vi "MainServer.vi"() -> ()   [LabVIEW 2012]
uses:
  <vilib>/addons/database/Connection.llb/DB Tools Open Connec (Path).vi
  <vilib>/addons/database/NI_Database_API.lvlib
panel:
  out "error":i32[](array[numeric])
  out "length":i32[](array[numeric])
  in  "Port":u16=1721
  out "# of Connections":i32
  in  "stop":bool
  in  "listen halted":bool
  out "Array":string[](array[string])
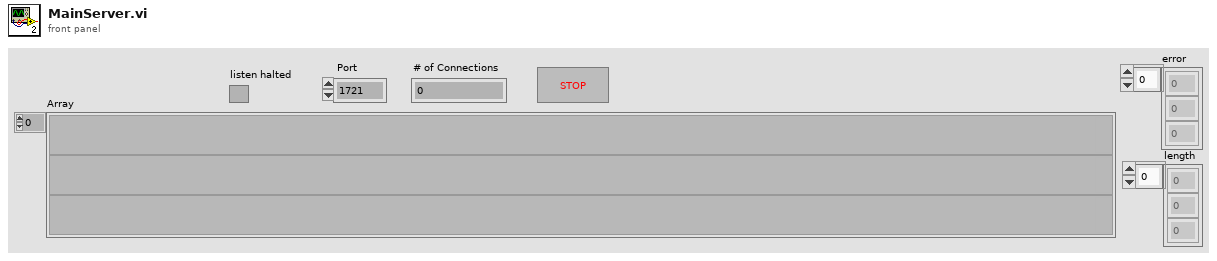
[diagram p1: front panel]
types:
  T1 = typedef "NI_Database_API.lvlib/Conn ObjectReference.ctl" = refnum<k1>
  T2 = enum16{"Standard", "Buffered", "CRLF", "Immediate"}
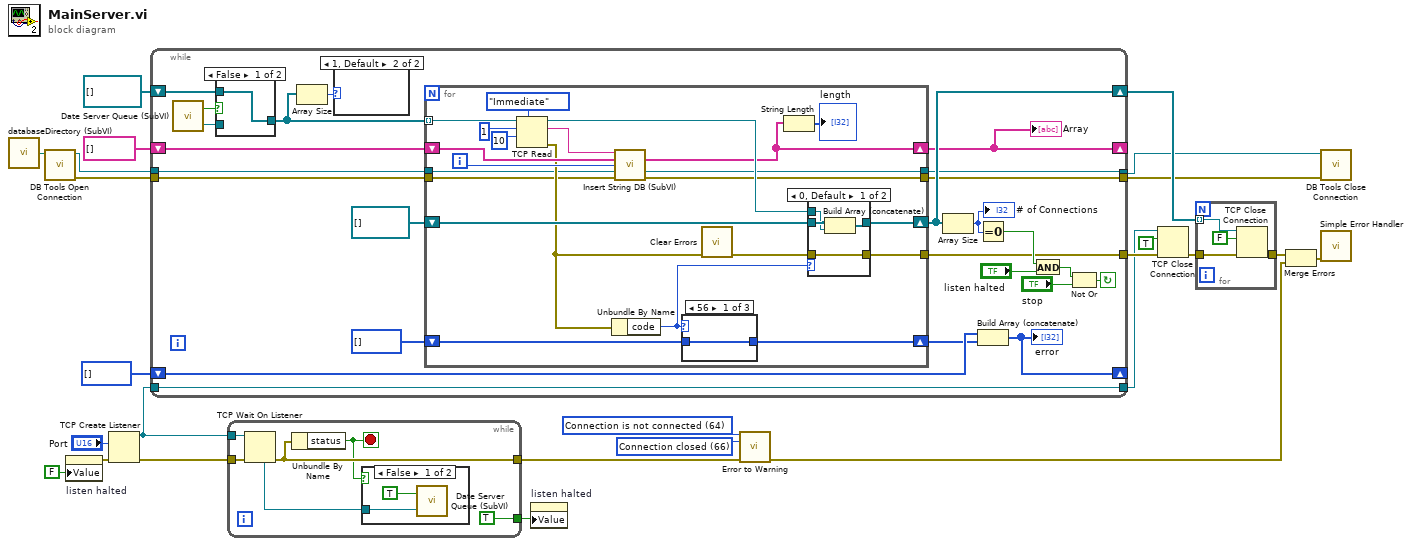
[diagram p0: block diagram]
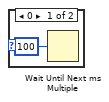
[diagram p2: hidden frame]
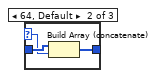
[diagram p3: hidden frame]
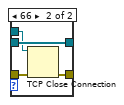
[diagram p5: hidden frame]
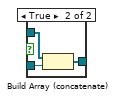
[diagram p6: hidden frame]
diagram:
  w18 = 66 items=["No Error", "Argument Error", "Memory Full", "Out of Zone", "End of File", "File Already Open", "Generic File IO Error", "File Not Found", "File Permission Error", "Disk Full", "Duplicate Path", "Too Many Files Open", "Not Enabled", "Resource File Not Found", "Cannot Add Resource", "Resource Not Found", "Image Not Found", "Image Memory Error", "Pen Does Not Exist", "Config Bad Type", "Config Token Not Found", "Config Parse Error", "Config Memory Error", "Bad External Code Format", "Bad External Code Offset", "External Code Not Present", "Null Window", "Destroy Window Mixup", "Null Menu", "Print Aborted", "Bad Print Record", "Print Driver Error", "Windows Error During Print", "Memory Error During Print", "Print Dialog Error", "Generic Print Error", "Invalid Device Refnum", "Device Not Found", "Device Parameter Error", "Device Unit Error", "Can't Open Device", "Device Call Aborted", "Generic Error", "Cancelled By User", "Object ID Too Low", "Object ID Too High", "Object Not In Heap", "Unknown Heap", "Bad DefProc ID", "DefProc Not In Table", "Message Out Of Range", "Null Method", "Unknown Message", "Manager Call Not Supported", "Bad address", "Connection In progress", "Connection timed out", "Connection is already in progress", "Network attribute not supported", "Network error", "Address in use", "System out of memory", "Connection aborted", "Connection refused", "Connection is not connected", "Connection is already connected", "Connection closed", "Initialize error (interapplication manager)", "Bad occurrence", "Wait on unbound occurrence handler", "Occurrence queue overflow", "Bad path", "Semaphore not signaled", "Unrecognized type (interapplication manager)"] ("2nd Error to Convert")
  w19 = 64 items=["No Error", "Argument Error", "Memory Full", "Out of Zone", "End of File", "File Already Open", "Generic File IO Error", "File Not Found", "File Permission Error", "Disk Full", "Duplicate Path", "Too Many Files Open", "Not Enabled", "Resource File Not Found", "Cannot Add Resource", "Resource Not Found", "Image Not Found", "Image Memory Error", "Pen Does Not Exist", "Config Bad Type", "Config Token Not Found", "Config Parse Error", "Config Memory Error", "Bad External Code Format", "Bad External Code Offset", "External Code Not Present", "Null Window", "Destroy Window Mixup", "Null Menu", "Print Aborted", "Bad Print Record", "Print Driver Error", "Windows Error During Print", "Memory Error During Print", "Print Dialog Error", "Generic Print Error", "Invalid Device Refnum", "Device Not Found", "Device Parameter Error", "Device Unit Error", "Can't Open Device", "Device Call Aborted", "Generic Error", "Cancelled By User", "Object ID Too Low", "Object ID Too High", "Object Not In Heap", "Unknown Heap", "Bad DefProc ID", "DefProc Not In Table", "Message Out Of Range", "Null Method", "Unknown Message", "Manager Call Not Supported", "Bad address", "Connection In progress", "Connection timed out", "Connection is already in progress", "Network attribute not supported", "Network error", "Address in use", "System out of memory", "Connection aborted", "Connection refused", "Connection is not connected", "Connection is already connected", "Connection closed", "Initialize error (interapplication manager)", "Bad occurrence", "Wait on unbound occurrence handler", "Occurrence queue overflow", "Bad path", "Semaphore not signaled", "Unrecognized type (interapplication manager)"] ("1st Error to Convert")
  n1 = call "databaseDirectory (SubVI).vi"() -> ("Application Directory"=w1:path)  [unwired: 1 in]
  n2 = call-poly <vilib>:"DB Tools Open Connection.vi"("connection information"=w1) -> ("error out"=w4:errorcluster, "connection reference"=w5:T1)  [unwired: 7 in]
  n3 = property on="listen halted" class="Bool (strict)"("Value"=FALSE) -> (error out=w14:errorcluster)  [unwired: 2 in, 1 out]
  n4 = TCP Create Listener(8:w14, 10:"Port") -> (0:w23:errorcluster, 3:w22:refnum<k5>)  [unwired: 4 out]
  n5 = while {
    shift-left: refnum<k5>[] [] ("empty") -> [w48]
    shift-right: [w46] -> w25
    tunnel: w22 -> [w39]
    tunnel: [w39] -> w7
    tunnel: [w38] -> w13
    shift-right: [w36] -> _
    shift-left: string[] [] -> [w37]
    shift-right: [w32] -> _
    shift-left: i32[] [] -> [w33]
    tunnel: w5 -> [w29]
    tunnel: w4 -> [w28]
    tunnel: [w27] -> w3
    tunnel: [w26] -> w2
    stop <- w41 continue-if-true
    n6 = call "Date Server Queue (SubVI).vi"() -> ("value"=w50:refnum<k5>, "valid?"=w49:bool)  [unwired: 2 in]
    n7 = case shown="False" w49 {
      tunnel: w50 -> [_ w90]
      tunnel: w48 -> [w87 w89]
      tunnel: [w87 w88] -> w34
      frame False {
      }
      frame True {
        n8 = Build Array (concatenate)(w89, w90) -> (w88:refnum<k5>[])
      }
    }
    n9 = Array Size(array=w34) -> (size(s)=w35:i32)
    n10 = case shown="1, Default" w35 {
      frame 0 {
        n11 = Wait Until Next ms Multiple(millisecond multiple=u32 100) -> ()  [unwired: 1 out]
      }
      frame 1, Default {
      }
    }
    n12 = for {
      tunnel: w34 -> [w69] mode=indexing
      shift-right: [w72] -> w46
      shift-left: refnum<k5>[] [] ("empty 2") -> [w73]
      tunnel: [w64] -> w38
      shift-right: [w62] -> w36
      shift-left: w37 -> [w67]
      shift-right: [w57] -> w30
      shift-left: i32[] [] -> [w58]
      tunnel: w29 -> [w56]
      tunnel: w28 -> [w55]
      tunnel: [w54] -> w27
      tunnel: [w53] -> w26
      i -> [w66]
      n13 = TCP Read(connection ID=w69, bytes to read=1, 7:T2."Immediate" ("mode (standard)"), 9:10) -> (connection ID out=w65:refnum<k5>, data out=w68:string, error out=w60:errorcluster)  [unwired: 1 in]
      n14 = Unbundle By Name(w60) -> ("code"=w59:i32)
      n15 = call "Insert String DB (SubVI).vi"("String Insert"=w68, "Array"=w67, "index"=w66, "Refnum in"=w56, "error in"=w55) -> ("output array"=w62:string[], "Refnum in 2"=w54:T1, "error out"=w53:errorcluster)  [unwired: 8 in]
      n16 = case shown="56" w59 {
        selector: w59 -> [_ w76 _]
        tunnel: w58 -> [w74 w77 w78]
        tunnel: [w74 w75 w78] -> w57
        frame 56 {
        }
        frame 64, Default {
          n17 = Build Array (concatenate)(w77, w76) -> (w75:i32[])
        }
        frame 0 {
        }
      }
      n18 = call <vilib>:"Clear Errors.vi"("error in (no error)"=w60) -> ("error out"=w63:errorcluster)  [unwired: 6 out]
      n19 = String Length(string=w62) -> (length=→"length":i32[])
      n20 = case shown="0, Default" w59 {
        tunnel: w73 -> [w82 w86]
        tunnel: [w81 w86] -> w72
        tunnel: w65 -> [w80 w83]
        tunnel: [w79 w84] -> w64
        tunnel: w63 -> [w79 w85]
        frame 0, Default {
          n21 = Build Array (concatenate)(w82, w80) -> (w81:refnum<k5>[])
        }
        frame 66 {
          n22 = TCP Close Connection(connection ID=w83, error in (no error)=w85) -> (error out=w84:errorcluster)  [unwired: 1 in, 1 out]
        }
      }
    }
    "Array" <- w36
    n23 = Array Size(array=w46) -> (size(s)=w44:i32)
    "# of Connections" <- w44
    n24 = Equal To 0?(x=w44) -> (x = 0?=w45:bool)
    n25 = Build Array (concatenate)(w33, w30) -> (w32:i32[])
    "error" <- w32
    n26 = And(x=w45, y="listen halted") -> (x .and. y?=w42:bool)
    n27 = Not Or(1:"stop", 2:w42) -> (0:w41:bool)
  }
  n28 = while "Listen loop.  Append new connections to a synchronized queue." {
    tunnel: w22 -> [w95]
    tunnel: w23 -> [w96]
    tunnel: [w93] -> w20
    tunnel: [TRUE] -> w21
    stop <- w92 stop-if-true
    n29 = TCP Wait On Listener(8:w96, 11:w95) -> (0:w93:errorcluster, 4:w94:refnum<k5>)  [unwired: 5 out]
    n30 = Unbundle By Name(w93) -> ("status"=w92:bool)
    n31 = case shown="False" w92 {
      tunnel: w94 -> [w97 _]
      frame False {
        n32 = call "Date Server Queue (SubVI).vi"("new value"=w97, "set queue? (F: de-queue)"=TRUE) -> ()  [unwired: 2 out]
      }
      frame True {
      }
    }
  }
  n33 = property on="listen halted" class="Bool (strict)"("Value"=w21) -> ()  [unwired: 2 in, 2 out]
  n34 = call <vilib>:"Error to Warning.vi"("1st Error to Convert"=w19, "2nd Error to Convert"=w18, "error in"=w20) -> ("warning out"=w11:errorcluster)  [unwired: 2 in, 10 out]
  n35 = TCP Close Connection(connection ID=w7, abort (F)=TRUE, error in (no error)=w13) -> (error out=w12:errorcluster)  [unwired: 1 out]
  n36 = for {
    tunnel: w25 -> [w102] mode=indexing
    tunnel: [w101] -> w17
    tunnel: w12 -> [w100]
    n37 = TCP Close Connection(connection ID=w102, abort (F)=FALSE, error in (no error)=w100) -> (error out=w101:errorcluster)  [unwired: 1 out]
  }
  n38 = Merge Errors(w17, w11) -> (w16:errorcluster)
  n39 = call <vilib>:"DB Tools Close Connection.vi"("error in (no error)"=w2, "connection reference"=w3) -> ()  [unwired: 5 in, 1 out]
  n40 = call <vilib>:"Simple Error Handler.vi"("error in (no error)"=w16) -> ()  [unwired: 1 in, 8 out]
